vi "Set Register Data.vi"(8 "error in (no error)":errorcluster, 10 "Register Data":T1 format="%02x", 11 "RFFE Standard Command in":refnum<class "RFFE Standard Command.lvclass">) -> (0 "error out":errorcluster, 3 "RFFE Standard Command out":refnum<class "RFFE Standard Command.lvclass">)   [LabVIEW 2018, in "MIPI RFFE API.lvlib" / "RFFE Standard Command.lvclass"]
uses:
  RFFE Standard Command.lvclass
  Register Data.ctl
  RFFE Standard Command.lvclass/RFFE Standard Command.ctl
  MIPI RFFE API.lvlib
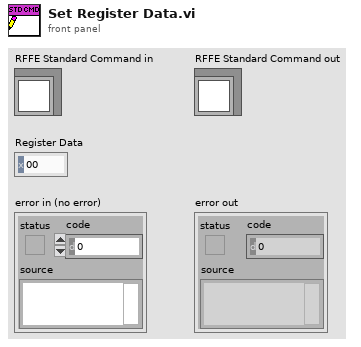
[diagram p1: front panel]
types:
  T1 = typedef "MIPI RFFE API.lvlib/Register Data.ctl" = u8
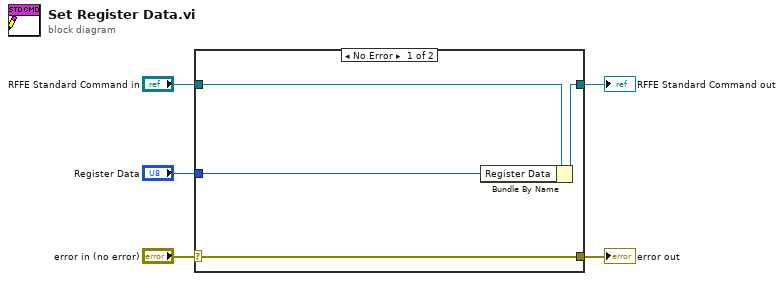
[diagram p0: block diagram]
diagram:
  n1 = case shown="No Error" "error in (no error)" {
    selector: "error in (no error)" -> [w9 w10]
    tunnel: [w9 w10] -> w4
    tunnel: [w7 w11] -> w2
    tunnel: "RFFE Standard Command in" -> [w8 w11]
    tunnel: "Register Data" -> [w6 _]
    frame No Error {
      n2 = Bundle By Name(cluster=w8, "Register Data"=w6) -> (w7:refnum<class "RFFE Standard Command.lvclass">)
    }
    frame Error {
    }
  }
  "error out" <- w4
  "RFFE Standard Command out" <- w2
